vi "ipg_ushort.vi"(1 "String":string) -> (0 "Ushort":u16)   [LabVIEW 2023, in "Laser_com_2022.lvlib"]
uses:
  Laser_com_2022.lvlib
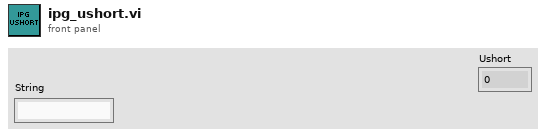
[diagram p1: front panel]
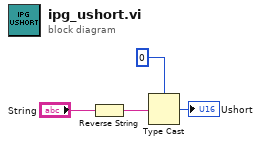
[diagram p0: block diagram]
diagram:
  n1 = Reverse String(1:"String") -> (0:w3:string)
  n2 = Type Cast(type=u16 0, x=w3) -> (*(type *) &x=→"Ushort":u16)
